vi "Reset.vi"(4 "error in (no error)":errorcluster, 7 "VISA resource name":refnum<visa-resource-name>) -> (0 "error out":errorcluster, 3 "VISA resource name out":refnum<visa-resource-name>)   [LabVIEW 2017, in "Newport ESP301.lvlib"]
doc: "This command is used to perform a hardware reset of the controller. It performs the following preliminary tasks before resetting the controller:\n1. Stop all the axes that are in motion. The deceleration value specified using the command AG is used to stop the axes.\n2. Wait for 500 ms to allow the axes to settle.\n3. Disable all the axes by turning the power OFF.\n4. Reset to the controller card.\nOnce the command to reset the controller is detected by the DSP, the controller will stay in reset for a minimum of 200 ms. After the reset condition has occurred (i.e., after the 200 ms reset time), the controller firmware reboots the controller. At this point, all the parameters last saved to the non-volatile flash memory on the controller will be restored. Furthermore, the controller will detect any stages (ESP compatible or otherwise) and drivers connected to the controller. This process can take anywhere up to 20 seconds depending upon the controller configuration.\n<B>NOTE:</B> This command is affective only when the watchdog timer is enabled through appropriate jumper setting on the controller card (default factory setting is \"enabled\").\n<B>NOTE:</B> There are no reset for USB link."
uses:
  Newport ESP301.lvlib
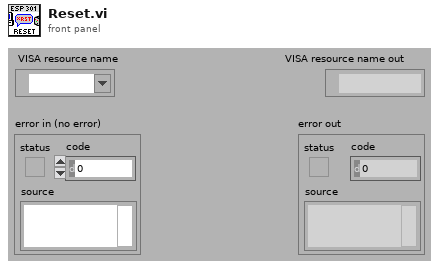
[diagram p1: front panel]
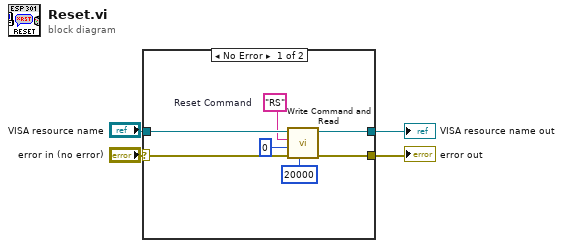
[diagram p0: block diagram]
diagram:
  n1 = case shown="No Error" "error in (no error)" {
    selector: "error in (no error)" -> [w8 w12]
    tunnel: [w5 w13] -> w4
    tunnel: [w6 w12] -> w3
    tunnel: "VISA resource name" -> [w11 w13]
    frame No Error {
      w10 = "RS"  # Reset Command
      n2 = call "Write Command and Read.vi"("Wait before read (0ms)"=u32 20000, "error in (no error)"=w8, "Bytes to read (100)"=u32 0, "Command"=w10, "VISA resource name"=w11) -> ("error out"=w6:errorcluster, "VISA resource name out"=w5:refnum<visa-resource-name>)  [unwired: 2 in, 1 out]
    }
    frame Error {
    }
  }
  "error out" <- w3
  "VISA resource name out" <- w4
